vi "Check and Override Channel Configuration.vi"(8 "error in (no error)":errorcluster, 10 "Custom Config Data in":u8[](array[numeric]) format="%.0x", 11 "CIF_CIPC_Chn_String in":refnum<class "CIF_CIPC_Chn_String.lvclass">) -> (0 "error out":errorcluster, 2 "Custom Config Data out":u8[](array[numeric]) format="%.0x", 3 "CIF_CIPC_Chn_String out":refnum<class "CIF_CIPC_Chn_String.lvclass">)   [LabVIEW 2021, in "CIF_CIPC_Chn_String.lvclass"]
uses:
  CIF_CIPC_Chn_String.lvclass
  CIF_CIPC_Chn_String.lvclass/CIF_CIPC_Chn_String.ctl
  ChannelCommon/ChannelCommon.lvlib
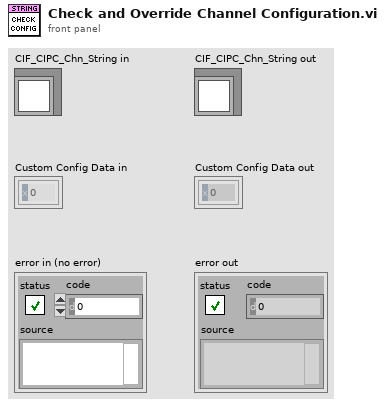
[diagram p1: front panel]
types:
  T1 = typedef "ChannelCommon.lvlib/FIFO Config.ctl" = cluster{"Max Bytes/Msg":u64, "Max Msg/FIFO":u64, "Flags":u64, "Custom Data":u8[]}
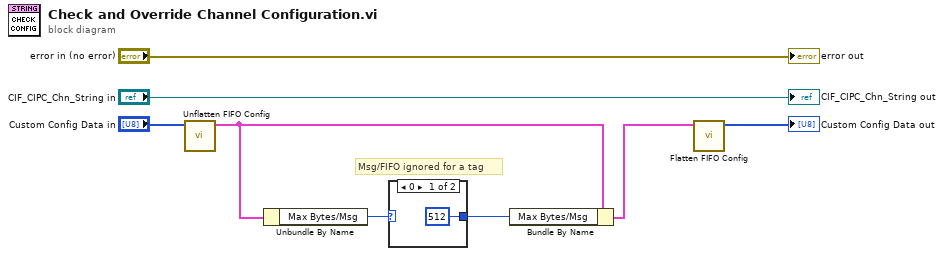
[diagram p0: block diagram]
diagram:
  # "Msg/FIFO ignored for a tag"
  n1 = call "Unflatten FIFO Config.vi"("Flattened Data in"="Custom Config Data in") -> ("FIFO Config out"=w3:T1)  [unwired: 9 in, 1 out]
  n2 = Unbundle By Name(w3) -> ("Max Bytes/Msg"=w4:u64)
  n3 = case shown="0" w4 {
    selector: w4 -> [_ w10]
    tunnel: [u64 512 ("y") w10] -> w1
    frame 0 {
    }
    frame 1, Default {
    }
  }
  n4 = Bundle By Name(cluster=w3, "Max Bytes/Msg"=w1) -> (w2:T1)
  n5 = call "Flatten FIFO Config.vi"("FIFO Config in"=w2) -> ("Flattened FIFO Config"=→"Custom Config Data out":u8[])  [unwired: 10 in]
  "error out" <- "error in (no error)"
  "CIF_CIPC_Chn_String out" <- "CIF_CIPC_Chn_String in"
